vi "Parse All Attributes.vi"(8 "error in":errorcluster, 11 "Node in":refnum<k20>) -> (0 "error out":errorcluster, 2 "Channel Data":T1, 3 "Node out":refnum<k20>)   [LabVIEW 2024, in "Parser.lvlib" / "Channel.lvclass"]
uses:
  Channel.lvclass
  <vilib>/xml/Close Reference(Node).vi
  <resource>/objmgr/DOMUserDefRef.rc
  <vilib>/xml/NI_XML.lvlib
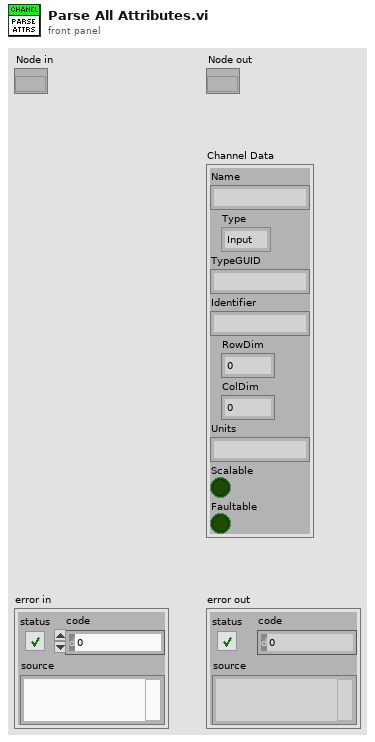
[diagram p1: front panel]
types:
  T1 = cluster{"Name":string, "Type":enum16{"Input", "Output"}, "TypeGUID":string, "Identifier":string, "RowDim":i32, "ColDim":i32, "Units":string, "Scalable":bool, "Faultable":bool}
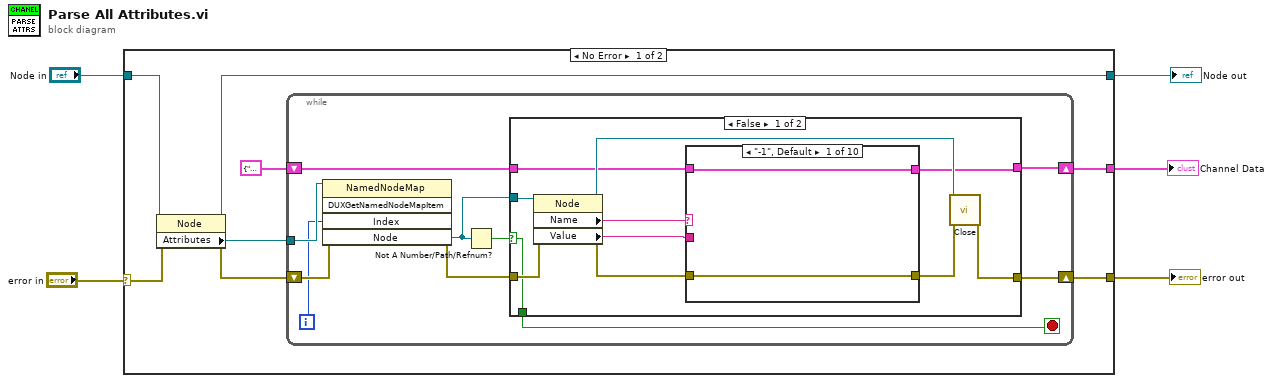
[diagram p0: block diagram]
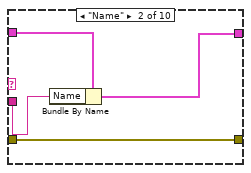
[diagram p2: hidden frame]
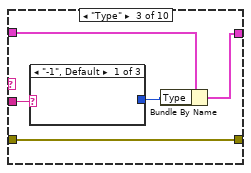
[diagram p3: hidden frame]
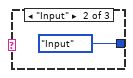
[diagram p4: hidden frame]
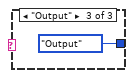
[diagram p5: hidden frame]
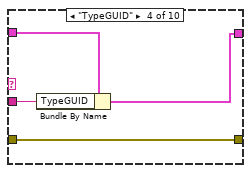
[diagram p6: hidden frame]
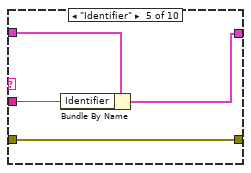
[diagram p7: hidden frame]
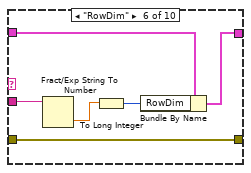
[diagram p8: hidden frame]
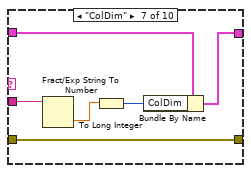
[diagram p9: hidden frame]
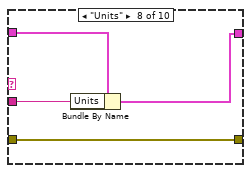
[diagram p10: hidden frame]
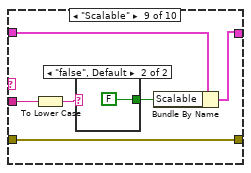
[diagram p11: hidden frame]
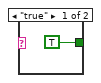
[diagram p12: hidden frame]
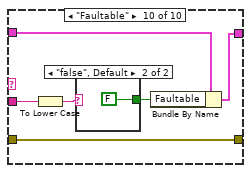
[diagram p13: hidden frame]
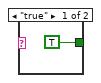
[diagram p14: hidden frame]
diagram:
  n1 = case shown="No Error" "error in" {
    selector: "error in" -> [w11 w92]
    tunnel: [w12 w92] -> w5
    tunnel: "Node in" -> [w10 w91]
    tunnel: [w7 w91] -> w2
    tunnel: [w6 _] -> w1
    frame No Error {
      n2 = property on="Property Node" class="Node"(reference=w10, error in=w11) -> (reference out=w7:refnum<k20>, error out=w13:errorcluster, "Attributes"=w9:refnum<k20>)
      n3 = while {
        tunnel: w9 -> [w20]
        shift-right: [w21] -> w12
        shift-left: w13 -> [w23]
        shift-right: [w14] -> w6
        shift-left: T1 {"Name"="", "Type"=enum."Input", "TypeGUID"="", "Identifier"="", "RowDim"=0, "ColDim"=0, "Units"="", "Scalable"=FALSE, "Faultable"=FALSE} ("Cluster of class private data") -> [w15]
        i -> [w18]
        stop <- w17 stop-if-true
        n4 = invoke on="Invoke Node" class="NamedNodeMap" method="DUXGetNamedNodeMapItem"(reference=w20, error in=w23, "Index"=w18) -> (error out=w22:errorcluster, "Node"=w16:refnum<k20>)  [unwired: 2 in, 3 out]
        n5 = Not A Number/Path/Refnum?(number/path/refnum=w16) -> (NaN/Path/Refnum?=w19:bool)
        n6 = case shown="False" w19 {
          selector: w19 -> [w28 w89]
          tunnel: w16 -> [w30 _]
          tunnel: w22 -> [w34 w90]
          tunnel: [w32 w90] -> w21
          tunnel: [w28 w89] -> w17
          tunnel: w15 -> [w25 w88]
          tunnel: [w24 w88] -> w14
          frame False {
            n7 = property on="Property Node" class="Node"(reference=w30, error in=w34) -> (reference out=w26:refnum<k20>, error out=w33:errorcluster, "Name"=w29:string, "Value"=w27:string)
            n8 = case shown="\"-1\", Default" w29 {
              tunnel: w27 -> [_ w39 w44 w50 w54 w60 w66 w70 w76 w84]
              tunnel: w33 -> [w36 w40 w45 w51 w55 w61 w67 w71 w77 w85]
              tunnel: w25 -> [w35 w38 w42 w49 w53 w57 w63 w69 w73 w81]
              tunnel: [w35 w37 w41 w48 w52 w56 w62 w68 w72 w80] -> w24
              tunnel: [w36 w40 w45 w51 w55 w61 w67 w71 w77 w85] -> w31
              frame "-1", Default {
              }
              frame "Name" {
                n9 = Bundle By Name(cluster=w38, "Name"=w39) -> (w37:T1)
              }
              frame "Type" {
                n10 = case shown="\"-1\", Default" w44 {
                  tunnel: [_ enum16{"Input", "Output"}."Input" enum16{"Input", "Output"}."Output"] -> w43
                  frame "-1", Default {
                  }
                  frame "Input" {
                  }
                  frame "Output" {
                  }
                }
                n11 = Bundle By Name(cluster=w42, "Type"=w43) -> (w41:T1)
              }
              frame "TypeGUID" {
                n12 = Bundle By Name(cluster=w49, "TypeGUID"=w50) -> (w48:T1)
              }
              frame "Identifier" {
                n13 = Bundle By Name(cluster=w53, "Identifier"=w54) -> (w52:T1)
              }
              frame "RowDim" {
                n14 = Fract/Exp String To Number(string=w60) -> (number=w58:dbl)  [unwired: 3 in, 1 out]
                n15 = To Long Integer(number=w58) -> (32bit integer=w59:i32)
                n16 = Bundle By Name(cluster=w57, "RowDim"=w59) -> (w56:T1)
              }
              frame "ColDim" {
                n17 = Fract/Exp String To Number(string=w66) -> (number=w64:dbl)  [unwired: 3 in, 1 out]
                n18 = To Long Integer(number=w64) -> (32bit integer=w65:i32)
                n19 = Bundle By Name(cluster=w63, "ColDim"=w65) -> (w62:T1)
              }
              frame "Units" {
                n20 = Bundle By Name(cluster=w69, "Units"=w70) -> (w68:T1)
              }
              frame "Scalable" {
                n21 = To Lower Case(string=w76) -> (all lower case string=w75:string)
                n22 = case shown="\"false\", Default" w75 {
                  tunnel: [TRUE ("Scalability") FALSE ("Scalability")] -> w74
                  frame "true" {
                  }
                  frame "false", Default {
                  }
                }
                n23 = Bundle By Name(cluster=w73, "Scalable"=w74) -> (w72:T1)
              }
              frame "Faultable" {
                n24 = To Lower Case(string=w84) -> (all lower case string=w83:string)
                n25 = case shown="\"false\", Default" w83 {
                  tunnel: [TRUE ("Scalability") FALSE ("Scalability")] -> w82
                  frame "true" {
                  }
                  frame "false", Default {
                  }
                }
                n26 = Bundle By Name(cluster=w81, "Faultable"=w82) -> (w80:T1)
              }
            }
            n27 = call-poly <vilib>:"Close.vi"("error in (no error)"=w31, "node"=w26) -> ("error out"=w32:errorcluster)  [unwired: 7 in]
          }
          frame True {
          }
        }
      }
    }
    frame Error {
    }
  }
  "error out" <- w5
  "Node out" <- w2
  "Channel Data" <- w1
